vi "Block Read Iterator.vi"(8 "error in (no error)":errorcluster, 9 "Iterations (1000)":i32=110, 10 "Channel Count":i32, 11 "GE 5565PIORC in":refnum<class "GE 5565PIORC Old.lvclass">) -> (0 "error out":errorcluster, 1 "Histogram Graph":T1(graph), 2 "Metrics":T2 {"Transfer Rate" format="%.2pB/s"; "Duration Std. Dev." format="%.0f µs"; "Duration Average" format="%.0f µs"}, 3 "GE 5565PIORC out":refnum<class "GE 5565PIORC Old.lvclass">)   [LabVIEW 2016]
uses:
  Source/GE 5565PIORC/GE 5565PIORC Old.lvclass
  Controls/Throughput Metrics.ctl
  Source/GE 5565PIORC/GE 5565PIORC Old.lvclass/GE 5565PIORC Old.ctl
  Source/GE 5565PIORC/VIs/Binary Operations/Align to 8-byte Boundary.vi
  Source/GE 5565PIORC/VIs/Binary Operations/Align to 16-byte Boundary.vi
  Source/GE 5565PIORC/VIs/DMA/DMA.Transfer Size.vi
  Source/GE 5565PIORC/VIs/Registers/Local Configuration.PCI Address.Set.vi
  Source/GE 5565PIORC/VIs/Registers/Local Configuration.DMADPR0.First Descriptor Address.Set.vi
  Source/GE 5565PIORC/VIs/DMA/DMA.Scatter-Gather.Link Block Descriptors.vi
  Source/GE 5565PIORC/VIs/DMA/DMA.Scatter-Gather.Commit Blocks.vi
  Source/GE 5565PIORC/VIs/Registers/Local Configuration.Local Address.Set.vi
  Source/GE 5565PIORC/VIs/Registers/Local Configuration.Transfer Size.Set.vi
  Source/GE 5565PIORC/VIs/Registers/Local Configuration.DMADPR0.Transfer Direction.Set.vi
  Source/GE 5565PIORC/VIs/Registers/Local Configuration.DMAMODE0.Scatter-Gather Enable.Set.vi
  <vilib>/Utility/error.llb/Clear Errors.vi
  Source/GE 5565PIORC/VIs/Registers/Local Configuration.DMACSR0.DMA Start.Set.vi
  Source/GE 5565PIORC/VIs/Interrupts/Wait for PXI Interrupt Events.vi
  Source/GE 5565PIORC/VIs/Registers/Local Configuration.DMACSR0.DMA Clear Interrupt.Set.vi
  Source/GE 5565PIORC/VIs/Registers/Local Configuration.Get Register Offset.vi
  Source/GE 5565PIORC/VIs/Binary Operations/Set Bits.vi
  Source/GE 5565PIORC/VIs/Binary Operations/Set Bits U32.vi
  Source/GE 5565PIORC/VIs/Binary Operations/Get Bits.vi
  Source/GE 5565PIORC/VIs/Binary Operations/Get Bits U32.vi
  Source/GE 5565PIORC/VIs/DMA/DMA.Read Single.vi
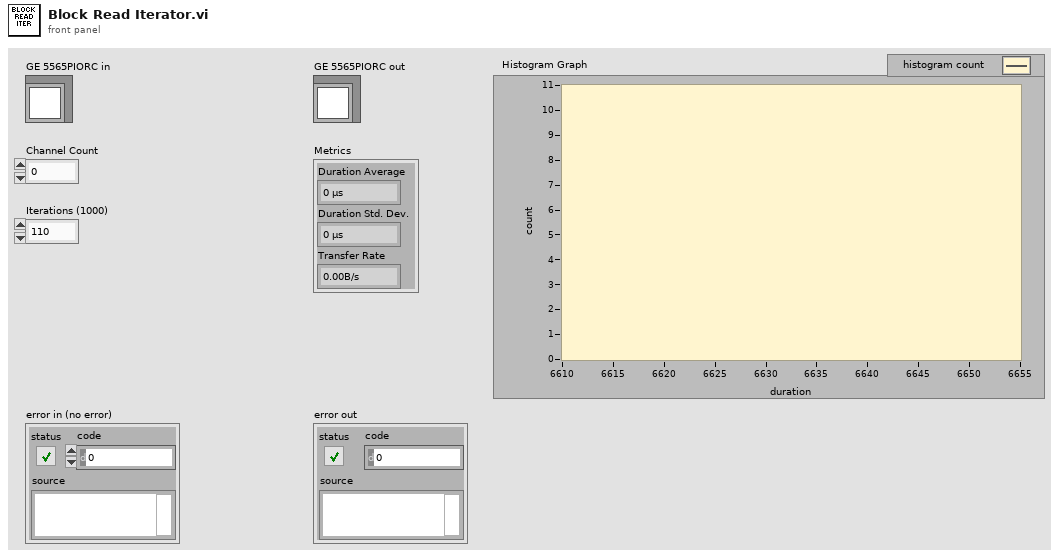
[diagram p1: front panel]
types:
  T1 = cluster{"X Values":dbl[], "Histogram: h(x)":i32[]}
  T2 = typedef "Throughput Metrics.ctl" = cluster{"Duration Average":u32, "Duration Std. Dev.":u32, "Transfer Rate":dbl}
  T3 = typedef "GE 5565PIORC Old.lvclass/DMA Block Descriptor.ctl" = cluster{"descriptor ptr (VISA)":u32, "descriptor size":u32, "descriptor ptr (aligned)":u32, "data ptr (lower)":u32, "data ptr (upper)":u32, "data size":u32, "next descriptor ptr":u32}
  T4 = typedef "GE 5565PIORC Old.lvclass/DMA Transfer Spec.ctl" = cluster{"RFM Address":u32, "Block Descriptors":T3[]}
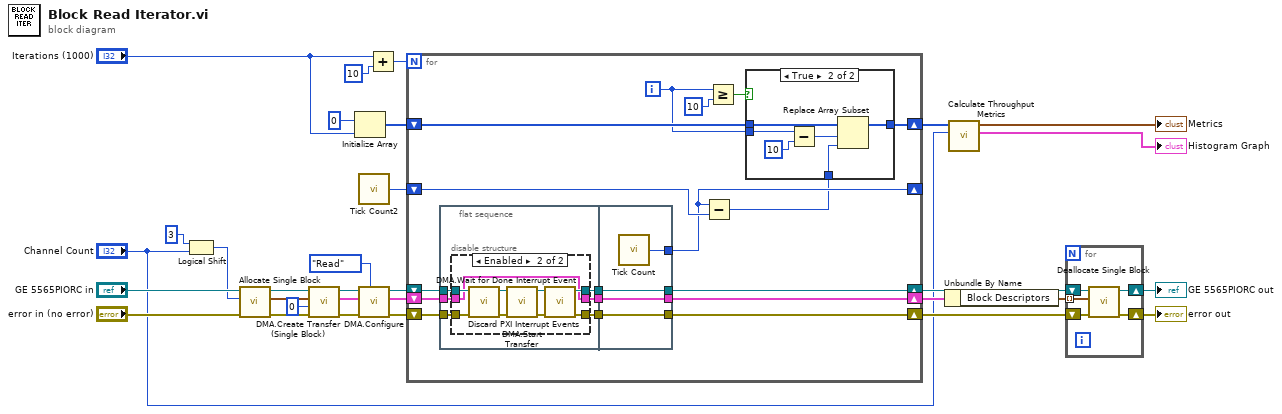
[diagram p0: block diagram]
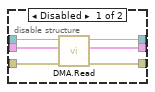
[diagram p3: hidden frame]
diagram:
  n1 = Logical Shift(y=i16 3, x="Channel Count") -> (x << y=w18:i32)
  n2 = call "Allocate Single Block.vi"("error in (no error)"="error in (no error)", "size (bytes)"=w18, "GE 5565PIORC in"="GE 5565PIORC in") -> ("error out"=w20:errorcluster, "Block Descriptor"=w17:T3, "GE 5565PIORC out"=w19:refnum<class "GE 5565PIORC Old.lvclass">)  [unwired: 6 in]
  n3 = call "DMA.Create Transfer (Single Block).vi"("error in (no error)"=w20, "RFM Offset"=u32 0, "Block Descriptor"=w17, "GE 5565PIORC in"=w19) -> ("error out"=w6:errorcluster, "DMA Transfer Spec"=w3:T4, "GE 5565PIORC out"=w7:refnum<class "GE 5565PIORC Old.lvclass">)  [unwired: 4 in, 1 out]
  n4 = Initialize Array(u32 0 ("x-y"), "Iterations (1000)") -> (w14:u32[])
  n5 = call "Tick Count2"() -> ("Tick Count(uSec)"=w24:u32)
  n6 = call "DMA.Configure.vi"("Transfer Direction"=enum16{"Write", "Read"}."Read", "error in (no error)"=w6, "DMA Transfer Spec"=w3, "GE 5565PIORC"=w7) -> ("error out"=w5:errorcluster, "DMA Transfer Spec out"=w2:T4, "GE 5565PIORC out"=w4:refnum<class "GE 5565PIORC Old.lvclass">)  [unwired: 5 in]
  n7 = Add(x="Iterations (1000)", y=10) -> (x+y=w31:i32)
  n8 = for {
    N: w31 -> [_]
    shift-right: [w39] -> _
    shift-left: w24 -> [w40]
    shift-right: [w42] -> w25
    shift-left: w4 -> [w48]
    shift-right: [w41] -> w26
    shift-left: w5 -> [w47]
    shift-right: [w37] -> w11
    shift-left: w14 -> [w38]
    shift-right: [w32] -> w13
    shift-left: w2 -> [w46]
    i -> [w35]
    n9 = flat-sequence {
      tunnel: w48 -> [w61]
      tunnel: w47 -> [w60]
      tunnel: w46 -> [w59]
      tunnel: [w57] -> w45
      tunnel: [w56] -> w44
      tunnel: [w58] -> w33
      tunnel: [w80] -> w42
      tunnel: w45 -> [w80]
      tunnel: w44 -> [w79]
      tunnel: [w79] -> w41
      tunnel: [w78] -> w39
      tunnel: w33 -> [w77]
      tunnel: [w77] -> w32
      frame #0 {
        n10 = disable-structure shown="Enabled" {
          disable-tunnel: w61 -> [w67 w74]
          disable-tunnel: w60 -> [w66 w73]
          disable-tunnel: w59 -> [w65 w68]
          disable-tunnel: [w64 w68] -> w58
          disable-tunnel: [w63 w72] -> w57
          disable-tunnel: [w62 w71] -> w56
          frame Disabled {
            n11 = call-poly "DMA.Read.vi"("error in (no error)"=w66, "DMA Transfer Spec"=w65, "GE 5565PIORC"=w67) -> ("error out"=w62:errorcluster, "DMA Transfer Spec out"=w64:T4, "GE 5565PIORC out"=w63:refnum<class "GE 5565PIORC Old.lvclass">)  [unwired: 5 in, 1 out]
          }
          frame Enabled {
            n12 = call "Discard PXI Interrupt Events.vi"("error in (no error)"=w73, "GE 5565PIORC in"=w74) -> ("error out"=w76:errorcluster, "GE 5565PIORC out"=w69:refnum<class "GE 5565PIORC Old.lvclass">)  [unwired: 8 in]
            n13 = call "DMA.Start Transfer.vi"("error in (no error)"=w76, "GE 5565PIORC"=w69) -> ("error out"=w75:errorcluster, "GE 5565PIORC out"=w70:refnum<class "GE 5565PIORC Old.lvclass">)  [unwired: 8 in]
            n14 = call "DMA.Wait for Done Interrupt Event.vi"("error in (no error)"=w75, "GE 5565PIORC"=w70) -> ("error out"=w71:errorcluster, "GE 5565PIORC out"=w72:refnum<class "GE 5565PIORC Old.lvclass">)  [unwired: 7 in, 1 out]
          }
        }
      }
      frame #1 {
        n15 = call "Tick Count"() -> ("Tick Count(uSec)"=w78:u32)
      }
    }
    n16 = Subtract(x=w39, y=w40) -> (x-y=w34:u32)
    n17 = Greater Or Equal?(x=w35, y=10) -> (x >= y?=w36:bool)
    n18 = case shown="True" w36 {
      tunnel: w38 -> [w49 w55]
      tunnel: [w49 w54] -> w37
      tunnel: w35 -> [_ w53]
      tunnel: w34 -> [_ w50]
      frame False {
      }
      frame True {
        n19 = Subtract(x=w53, y=10) -> (x-y=w51:i32)
        n20 = Replace Array Subset(array=w55, new element=w50, index=w51) -> (w54:u32[])
      }
    }
  }
  n21 = Unbundle By Name(w13) -> ("Block Descriptors"=w12:T3[])
  n22 = call "Calculate Throughput Metrics.vi"("Channel Count"="Channel Count", "Durations"=w11) -> ("Histogram Graph"=→"Histogram Graph":T1, "Metrics"=→"Metrics":T2)  [unwired: 8 in]
  n23 = for {
    tunnel: w12 -> [w81] mode=indexing
    shift-right: [w85] -> w28
    shift-left: w26 -> [w83]
    shift-right: [w84] -> w27
    shift-left: w25 -> [w82]
    n24 = call "Deallocate Single Block.vi"("error in (no error)"=w83, "Block Descriptor"=w81, "GE 5565PIORC in"=w82) -> ("error out"=w85:errorcluster, "GE 5565PIORC out"=w84:refnum<class "GE 5565PIORC Old.lvclass">)  [unwired: 7 in]
  }
  "error out" <- w28
  "GE 5565PIORC out" <- w27
